vi "FGV_Analog Input.vi"(7 "Command":T2, 8 "error in":errorcluster, 9 "Save data?":bool, 10 "Daq_ai_para":T1={"Channel"=[], "Sample rate"=0.0, "input terminal configuration"=-1} {"input terminal configuration" items=["Default"=-1, "RSE"=10083, "NRSE"=10078, "Differential"=10106, "Pseudodifferential"=12529]}, 11 "TDMS File Path":path) -> (0 "error out":errorcluster, 1 "Actual Sample Rate":dbl=1000.0 format="%0.2f", 2 "data":waveform(dbl)[](array[waveform]))   [LabVIEW 2017]
uses:
  Command.ctl
  <vilib>/DAQmx/read.llb/DAQmx Read (Analog 1D Wfm NChan NSamp).vi
  <vilib>/DAQmx/create/channels.llb/DAQmx Create Channel (AI-Voltage-Basic).vi
  <vilib>/DAQmx/configure/timing.llb/DAQmx Timing (Sample Clock).vi
  <vilib>/DAQmx/configure/task.llb/DAQmx Configure Logging (TDMS).vi
  <vilib>/DAQmx/miscellaneous.llb/DAQmx Fill In Error Info.vi
  <resource>/objmgr/daqmx.rc
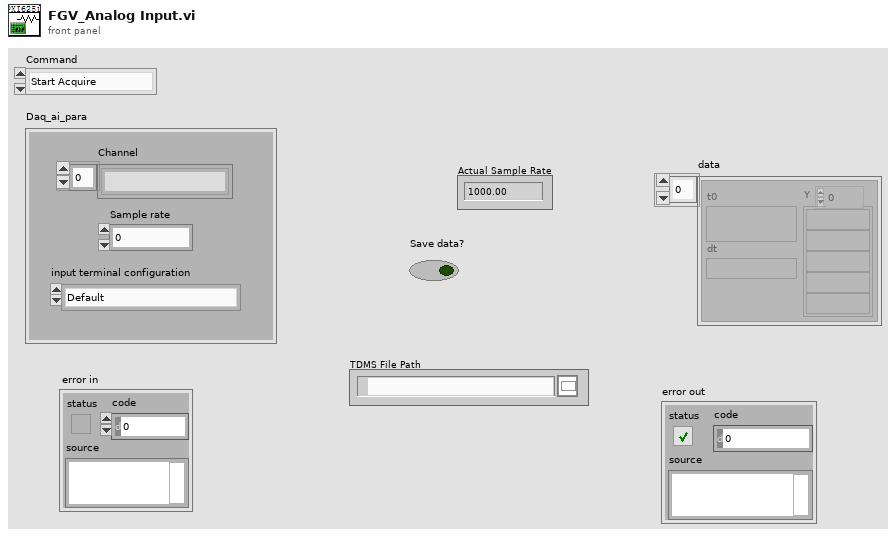
[diagram p1: front panel]
types:
  T1 = cluster{"Channel":string[], "Sample rate":dbl, "input terminal configuration":i32}
  T2 = typedef "Command.ctl" = enum16{"Start Acquire", "Read Data", "Release task"}
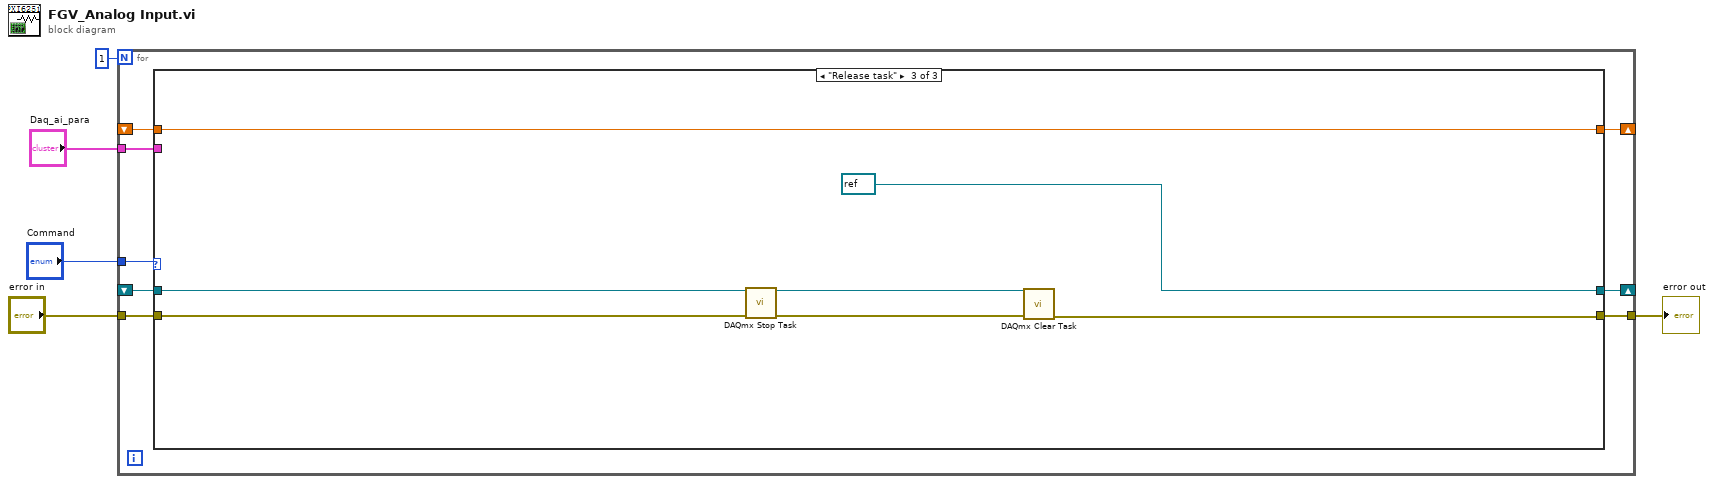
[diagram p0: block diagram]
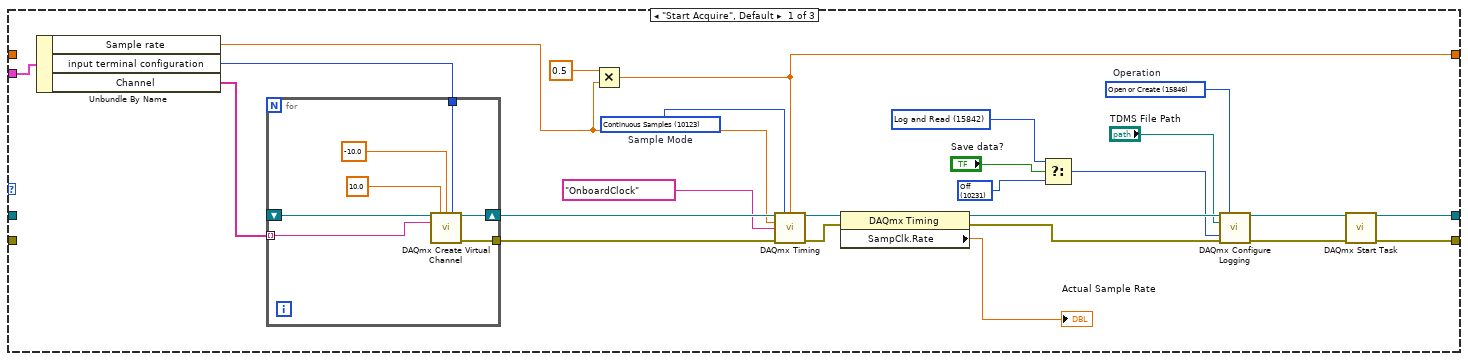
[diagram p2: hidden frame]
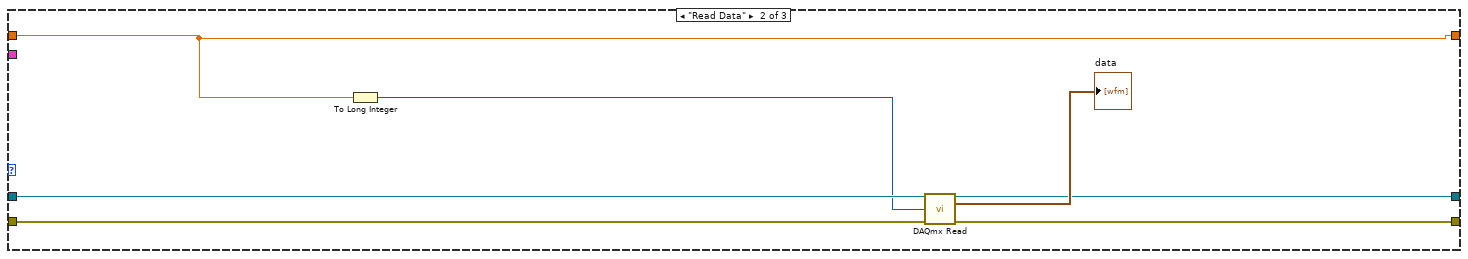
[diagram p3: hidden frame]
diagram:
  n1 = for {
    N: 1 -> [_]
    tunnel: "Command" -> [w13]
    tunnel: "error in" -> [w12]
    tunnel: [w11] -> w1
    shift-right: [w10] -> _
    shift-left: _ -> [w9]
    tunnel: "Daq_ai_para" -> [w8]
    shift-right: [w7] -> _
    shift-left: _ -> [w6]
    n2 = case shown="\"Release task\"" w13 {
      tunnel: w12 -> [_ w51 w54]
      tunnel: [w15 w50 w58] -> w11
      tunnel: [w17 w48 refnum<k21> refnum ("task out")] -> w10
      tunnel: w9 -> [_ w52 w59]
      tunnel: w8 -> [w25 _ _]
      tunnel: [w14 w46 w53] -> w7
      tunnel: w6 -> [_ w46 w53]
      frame "Start Acquire", Default {
        w18 = 10231 items=["Off"=10231, "Log and Read"=15842] ("Logging Mode")
        w30 = 15842 items=["Off"=10231, "Log and Read"=15842] ("Logging Mode")
        w31 = 15846 items=["Open"=10437, "Open or Create"=15846, "Create or Replace"=15847, "Create"=15848]  # Operation
        w36 = 10123 items=["Finite Samples"=10178, "Continuous Samples"=10123, "Hardware Timed Single Point"=12522]  # Sample Mode
        n3 = Unbundle By Name(w25) -> ("Sample rate"=w22:dbl, "input terminal configuration"=w23:i32, "Channel"=w24:string[])
        n4 = for {
          tunnel: [w45] -> w35
          shift-right: [w44] -> w34
          shift-left: _ -> [w41]
          tunnel: w24 -> [w40] mode=indexing
          tunnel: w23 -> [w39]
          n5 = call-poly <vilib>:"DAQmx Create Virtual Channel.vi"("task in"=w41, "maximum value"=10.0 ("Max Voltage"), "minimum value"=-10.0 ("Min Voltage"), "input terminal configuration"=w39, "physical channels"=w40) -> ("task out"=w44:refnum<k21>, "error out"=w45:errorcluster)  [unwired: 9 in]
        }
        n6 = Multiply(x=0.5, y=w22) -> (x*y=w14:dbl)
        n7 = call-poly <vilib>:"DAQmx Timing.vi"("task/channels in"=w34, "sample mode"=w36, "samples per channel"=w14, "rate"=w22, "source"=tag "OnboardClock" ("Sample Clock Source"), "error in"=w35) -> ("task out"=w38:refnum<k21>, "error out"=w37:errorcluster)  [unwired: 8 in]
        n8 = property class="DAQmx Timing"(reference=w38, error in=w37) -> (reference out=w33:refnum<k21>, error out=w32:errorcluster, "SampClk.Rate"=→"Actual Sample Rate":dbl)
        n9 = Select(t=w30, s="Save data?", f=w18) -> (s? t:f=w20:i32)
        n10 = call-poly <vilib>:"DAQmx Configure Logging.vi"("task/channels in"=w33, "operation"=w31, "file path"="TDMS File Path", "logging mode"=w20, "error in"=w32) -> ("task out"=w21:refnum<k21>, "error out"=w16:errorcluster)  [unwired: 9 in]
        n11 = call <vilib>:"DAQmx Start Task.vi"("task/channels in"=w21, "error in"=w16) -> ("task out"=w17:refnum<k21>, "error out"=w15:errorcluster)  [unwired: 12 in]
      }
      frame "Read Data" {
        n12 = To Long Integer(number=w46) -> (32bit integer=w47:i32)
        n13 = call-poly <vilib>:"DAQmx Read.vi"("task/channels in"=w52, "number of samples per channel"=w47, "error in"=w51) -> ("task out"=w48:refnum<k21>, "data"=→"data":waveform(dbl)[], "error out"=w50:errorcluster)  [unwired: 10 in]
      }
      frame "Release task" {
        n14 = call <vilib>:"DAQmx Stop Task.vi"("task/channels in"=w59, "error in"=w54) -> ("task out"=w56:refnum<k21>, "error out"=w55:errorcluster)  [unwired: 12 in]
        n15 = call <vilib>:"DAQmx Clear Task.vi"("task in"=w56, "error in"=w55) -> ("error out"=w58:errorcluster)  [unwired: 13 in]
      }
    }
  }
  "error out" <- w1
